vi "簡易計算機.vi"() -> ()   [LabVIEW 2009]
panel:
  out "/ temp":bool
  out "X temp":bool
  out "- temp":bool
  out "+ temp":bool
  out "I_Temp":dbl
  in  "=":bool
  in  ".":bool
  in  "Sqrt":bool
  in  "/":bool
  in  "X":bool
  in  "-":bool
  in  "+":bool
  in  "9":bool
  in  "8":bool
  in  "7":bool
  in  "6":bool
  in  "5":bool
  in  "4":bool
  in  "stop":bool
  in  "C":bool
  in  "0":bool
  in  "3":bool
  in  "2":bool
  in  "1":bool
  out "String":string="0"
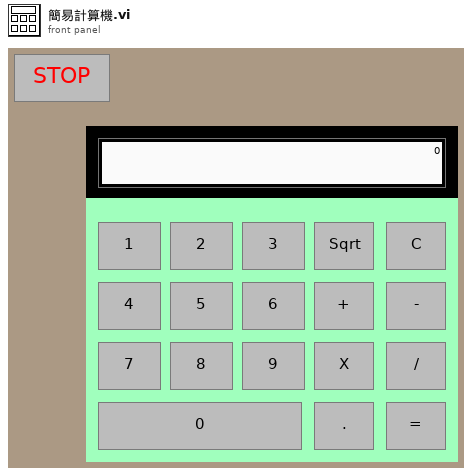
[diagram p1: front panel]
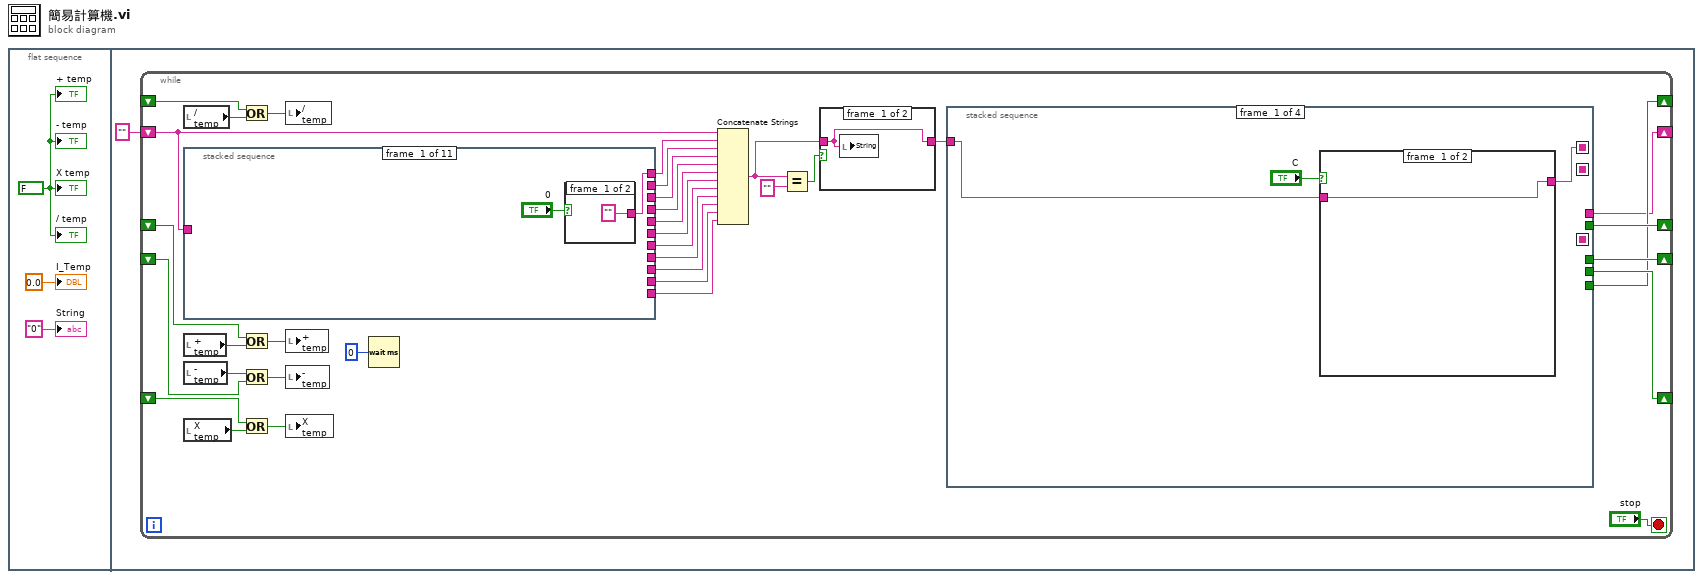
[diagram p0: block diagram]
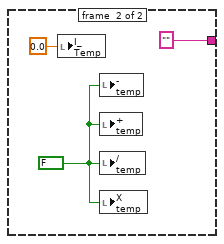
[diagram p2: hidden frame]
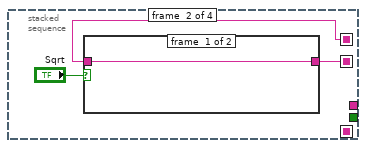
[diagram p3: hidden frame]
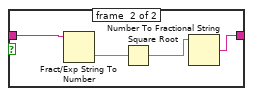
[diagram p4: hidden frame]
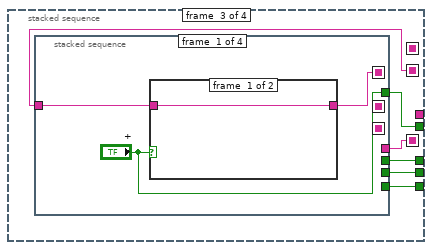
[diagram p5: hidden frame]
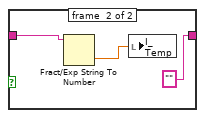
[diagram p6: hidden frame]
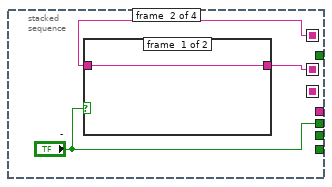
[diagram p7: hidden frame]
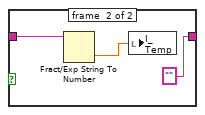
[diagram p8: hidden frame]
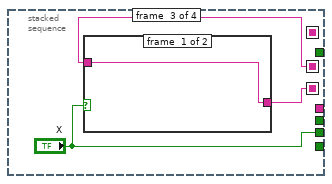
[diagram p9: hidden frame]
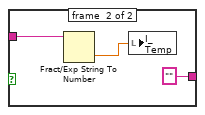
[diagram p10: hidden frame]
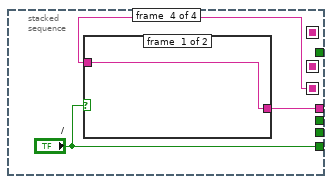
[diagram p11: hidden frame]
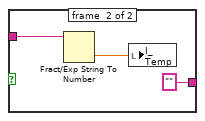
[diagram p12: hidden frame]
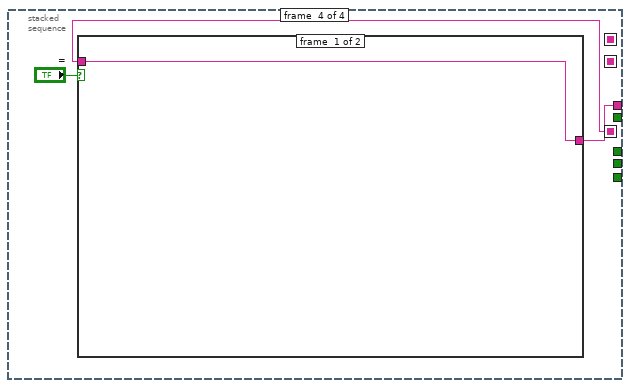
[diagram p13: hidden frame]
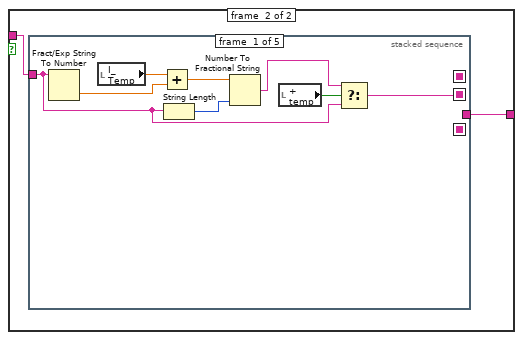
[diagram p14: hidden frame]
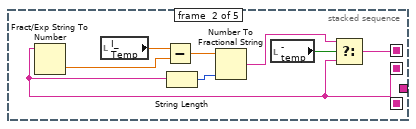
[diagram p15: hidden frame]
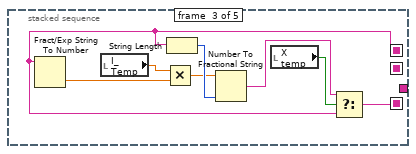
[diagram p16: hidden frame]
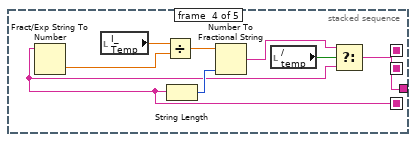
[diagram p17: hidden frame]
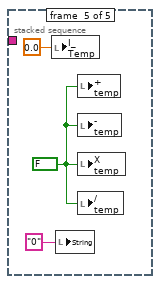
[diagram p18: hidden frame]
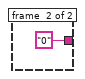
[diagram p19: hidden frame]
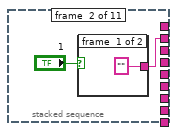
[diagram p20: hidden frame]
diagram:
  n1 = flat-sequence {
    frame #0 {
      w2 = FALSE
      "String" <- "0" ("String")
      "I_Temp" <- 0.0 ("Temp")
      "+ temp" <- w2
      "- temp" <- w2
      "X temp" <- w2
      "/ temp" <- w2
    }
    frame #1 {
      n2 = while {
        shift-right: [w5] -> _
        shift-left: "" ("String") -> [w24]
        shift-right: [w21] -> _
        shift-left: _ -> [w20]
        shift-right: [w18] -> _
        shift-left: _ -> [w17]
        shift-right: [w13] -> _
        shift-left: _ -> [w10]
        shift-right: [w12] -> _
        shift-left: _ -> [w11]
        stop <- "stop" stop-if-true
        n3 = local read "/ temp"() -> (w6:bool)
        n4 = stacked-sequence {
          tunnel: [w130 _ _ _ _ _ _ _ _ _ _] -> w37
          tunnel: [_ w134 _ _ _ _ _ _ _ _ _] -> w36
          tunnel: [_ _ w138 _ _ _ _ _ _ _ _] -> w35
          tunnel: [_ _ _ w142 _ _ _ _ _ _ _] -> w34
          tunnel: [_ _ _ _ w146 _ _ _ _ _ _] -> w33
          tunnel: [_ _ _ _ _ w150 _ _ _ _ _] -> w32
          tunnel: [_ _ _ _ _ _ w154 _ _ _ _] -> w31
          tunnel: [_ _ _ _ _ _ _ w158 _ _ _] -> w30
          tunnel: [_ _ _ _ _ _ _ _ w162 _ _] -> w29
          tunnel: [_ _ _ _ _ _ _ _ _ w166 _] -> w28
          tunnel: w24 -> [_ _ _ _ _ _ _ _ _ _ w171]
          tunnel: [_ _ _ _ _ _ _ _ _ _ w170] -> w22
          frame #0 {
            n5 = case shown="False" "0" {
              tunnel: ["" ("String") "0" ("String")] -> w130
              frame #0 {
              }
              frame #1 {
              }
            }
          }
          frame #1 {
            n6 = case shown="False" "1" {
              tunnel: ["" ("String") "1" ("String")] -> w134
              frame #0 {
              }
              frame #1 {
              }
            }
          }
          frame #2 {
            n7 = case shown="False" "2" {
              tunnel: ["" "2"] -> w138
              frame #0 {
              }
              frame #1 {
              }
            }
          }
          frame #3 {
            n8 = case shown="True" "3" {
              tunnel: ["" "3"] -> w142
              frame #0 {
              }
              frame #1 {
              }
            }
          }
          frame #4 {
            n9 = case shown="False" "4" {
              tunnel: ["" ("String") "4" ("String")] -> w146
              frame #0 {
              }
              frame #1 {
              }
            }
          }
          frame #5 {
            n10 = case shown="False" "5" {
              tunnel: ["" "5"] -> w150
              frame #0 {
              }
              frame #1 {
              }
            }
          }
          frame #6 {
            n11 = case shown="False" "6" {
              tunnel: ["" "6"] -> w154
              frame #0 {
              }
              frame #1 {
              }
            }
          }
          frame #7 {
            n12 = case shown="False" "7" {
              tunnel: ["" ("String") "7" ("String")] -> w158
              frame #0 {
              }
              frame #1 {
              }
            }
          }
          frame #8 {
            n13 = case shown="False" "8" {
              tunnel: ["" "8"] -> w162
              frame #0 {
              }
              frame #1 {
              }
            }
          }
          frame #9 {
            n14 = case shown="False" "9" {
              tunnel: ["" "9"] -> w166
              frame #0 {
              }
              frame #1 {
              }
            }
          }
          frame #10 {
            n15 = case shown="True" "." {
              tunnel: ["" w179] -> w170
              tunnel: w171 -> [_ w177]
              frame #0 {
              }
              frame #1 {
                w180 = "."
                n16 = Match Pattern(string=w177, regular expression=w180) -> (before substring=w176:string, after substring=w175:string)  [unwired: 3 out]
                n17 = Equal?(x=w177, y=w176) -> (x = y?=w182:bool)
                n18 = Equal?(x=w175, y=w180) -> (x = y?=w174:bool)
                n19 = Select(t="0.", s=w182, f=w180) -> (s? t:f=w178:string)
                n20 = Select(t=w176, s=w174, f=w178) -> (s? t:f=w179:string)
              }
            }
          }
        }
        n21 = local read "+ temp"() -> (w19:bool)
        n22 = local read "- temp"() -> (w16:bool)
        n23 = local read "X temp"() -> (w7:bool)
        n24 = Or(x=w11, y=w6) -> (x .or. y?=w9:bool)
        n25 = Or(x=w20, y=w19) -> (x .or. y?=w14:bool)
        n26 = Or(x=w16, y=w17) -> (x .or. y?=w15:bool)
        n27 = Or(x=w10, y=w7) -> (x .or. y?=w8:bool)
        n28 = local write "/ temp"(w9) -> ()
        n29 = local write "+ temp"(w14) -> ()
        n30 = local write "- temp"(w15) -> ()
        n31 = local write "X temp"(w8) -> ()
        n32 = Wait (ms)(milliseconds to wait=u32 0) -> ()  [unwired: 1 out]
        n33 = Concatenate Strings(w24, w37, w36, w35, w34, w33, w32, w31, w30, w29, w28, w22) -> (w27:string)
        n34 = Equal?(x=w27, y="") -> (x = y?=w25:bool)
        n35 = case shown="True" w25 {
          tunnel: w27 -> [w183 w184]
          tunnel: [w183 w184] -> w26
          frame #0 {
            n36 = local write "String"(w183) -> ()
          }
          frame #1 {
            n37 = local write "String"("0" ("String")) -> ()
          }
        }
        n38 = stacked-sequence {
          seq-local: [w40 _ _ _] -> [_ w48 _ _]
          seq-local: [_ w47 _ _] -> [_ _ w60 _]
          seq-local: [_ _ w56 _] -> [_ _ _ w91]
          tunnel: w26 -> [w41 _ _ _]
          tunnel: [_ _ w58 _] -> w21
          tunnel: [_ _ w59 _] -> w18
          tunnel: [_ _ w57 _] -> w13
          tunnel: [_ _ w55 _] -> w12
          tunnel: [_ _ _ w89] -> w5
          frame #0 {
            n39 = case shown="True" "C" {
              tunnel: w41 -> [w43 _]
              tunnel: [w43 "" ("String")] -> w40
              frame #0 {
              }
              frame #1 {
                w45 = FALSE
                n40 = local write "I_Temp"(0.0 ("Temp")) -> ()
                n41 = local write "- temp"(w45) -> ()
                n42 = local write "+ temp"(w45) -> ()
                n43 = local write "/ temp"(w45) -> ()
                n44 = local write "X temp"(w45) -> ()
              }
            }
          }
          frame #1 {
            n45 = case shown="True" "Sqrt" {
              tunnel: w48 -> [w50 w54]
              tunnel: [w50 w51] -> w47
              frame #0 {
              }
              frame #1 {
                n46 = Fract/Exp String To Number(string=w54) -> (number=w53:dbl)  [unwired: 4 out]
                n47 = Square Root(x=w53) -> (sqrt(x)=w52:dbl)
                n48 = Number To Fractional String(number=w52) -> (F-format string=w51:string)  [unwired: 3 out]
              }
            }
          }
          frame #2 {
            n49 = stacked-sequence {
              seq-local: [w61 _ _ _] -> [_ w69 _ _]
              seq-local: [_ w68 _ _] -> [_ _ w77 _]
              seq-local: [_ _ w76 _] -> [_ _ _ w84]
              tunnel: w60 -> [w63 _ _ _]
              tunnel: ["+" _ _ _] -> w58
              tunnel: [_ "-" _ _] -> w59
              tunnel: [_ _ "X" _] -> w57
              tunnel: [_ _ _ w83] -> w56
              tunnel: [_ _ _ "/"] -> w55
              frame #0 {
                n50 = case shown="True" "+" {
                  tunnel: w63 -> [w64 w67]
                  tunnel: [w64 "" ("String")] -> w61
                  frame #0 {
                  }
                  frame #1 {
                    n51 = Fract/Exp String To Number(string=w67) -> (number=w65:dbl)  [unwired: 4 out]
                    n52 = local write "I_Temp"(w65) -> ()
                  }
                }
              }
              frame #1 {
                n53 = case shown="True" "-" {
                  tunnel: w69 -> [w71 w74]
                  tunnel: [w71 ""] -> w68
                  frame #0 {
                  }
                  frame #1 {
                    n54 = Fract/Exp String To Number(string=w74) -> (number=w73:dbl)  [unwired: 4 out]
                    n55 = local write "I_Temp"(w73) -> ()
                  }
                }
              }
              frame #2 {
                n56 = case shown="True" "X" {
                  tunnel: w77 -> [w78 w81]
                  tunnel: [w78 "" ("String")] -> w76
                  frame #0 {
                  }
                  frame #1 {
                    n57 = Fract/Exp String To Number(string=w81) -> (number=w80:dbl)  [unwired: 4 out]
                    n58 = local write "I_Temp"(w80) -> ()
                  }
                }
              }
              frame #3 {
                n59 = case shown="True" "/" {
                  tunnel: w84 -> [w85 w88]
                  tunnel: [w85 "" ("String")] -> w83
                  frame #0 {
                  }
                  frame #1 {
                    n60 = Fract/Exp String To Number(string=w88) -> (number=w87:dbl)  [unwired: 4 out]
                    n61 = local write "I_Temp"(w87) -> ()
                  }
                }
              }
            }
          }
          frame #3 {
            n62 = case shown="True" "=" {
              tunnel: w91 -> [w92 w94]
              tunnel: [w92 w93] -> w89
              frame #0 {
              }
              frame #1 {
                n63 = stacked-sequence {
                  seq-local: [w100 _ _ _ _] -> [_ w106 _ _ _]
                  seq-local: [_ w105 _ _ _] -> [_ _ w113 _ _]
                  seq-local: [_ _ w114 _ _] -> [_ _ _ w123 _]
                  tunnel: w94 -> [w99 _ _ _ _]
                  tunnel: [_ _ _ w122 _] -> w93
                  frame #0 {
                    n64 = Fract/Exp String To Number(string=w99) -> (number=w97:dbl)  [unwired: 4 out]
                    n65 = local read "I_Temp"() -> (w98:dbl)
                    n66 = Add(x=w98, y=w97) -> (x+y=w95:dbl)
                    n67 = String Length(string=w99) -> (length=w101:i32)
                    n68 = Number To Fractional String(number=w95, precision (6)=w101) -> (F-format string=w102:string)  [unwired: 2 out]
                    n69 = local read "+ temp"() -> (w96:bool)
                    n70 = Select(t=w102, s=w96, f=w99) -> (s? t:f=w100:string)
                  }
                  frame #1 {
                    n71 = Fract/Exp String To Number(string=w106) -> (number=w110:dbl)  [unwired: 4 out]
                    n72 = local read "I_Temp"() -> (w108:dbl)
                    n73 = Subtract(x=w108, y=w110) -> (x-y=w103:dbl)
                    n74 = String Length(string=w106) -> (length=w109:i32)
                    n75 = Number To Fractional String(number=w103, precision (6)=w109) -> (F-format string=w107:string)  [unwired: 2 out]
                    n76 = local read "- temp"() -> (w104:bool)
                    n77 = Select(t=w107, s=w104, f=w106) -> (s? t:f=w105:string)
                  }
                  frame #2 {
                    n78 = Fract/Exp String To Number(string=w113) -> (number=w117:dbl)  [unwired: 4 out]
                    n79 = local read "I_Temp"() -> (w116:dbl)
                    n80 = Multiply(x=w116, y=w117) -> (x*y=w111:dbl)
                    n81 = String Length(string=w113) -> (length=w118:i32)
                    n82 = Number To Fractional String(number=w111, precision (6)=w118) -> (F-format string=w115:string)  [unwired: 2 out]
                    n83 = local read "X temp"() -> (w112:bool)
                    n84 = Select(t=w115, s=w112, f=w113) -> (s? t:f=w114:string)
                  }
                  frame #3 {
                    n85 = Fract/Exp String To Number(string=w123) -> (number=w125:dbl)  [unwired: 4 out]
                    n86 = local read "I_Temp"() -> (w121:dbl)
                    n87 = Divide(x=w121, y=w125) -> (x/y=w119:dbl)
                    n88 = String Length(string=w123) -> (length=w126:i32)
                    n89 = Number To Fractional String(number=w119, precision (6)=w126) -> (F-format string=w124:string)  [unwired: 2 out]
                    n90 = local read "/ temp"() -> (w120:bool)
                    n91 = Select(t=w124, s=w120, f=w123) -> (s? t:f=w122:string)
                  }
                  frame #4 {
                    w128 = FALSE ("+ temp")
                    n92 = local write "I_Temp"(0.0 ("I_Temp")) -> ()
                    n93 = local write "String"("0" ("String")) -> ()
                    n94 = local write "+ temp"(w128) -> ()
                    n95 = local write "- temp"(w128) -> ()
                    n96 = local write "X temp"(w128) -> ()
                    n97 = local write "/ temp"(w128) -> ()
                  }
                }
              }
            }
          }
        }
      }
    }
  }
